vi "Update SyncMethod Events.vi"(8 "error in (no error)":errorcluster, 11 "Server class in":refnum<vi>) -> (0 "error out":errorcluster, 3 "Server class out":refnum<vi>)   [LabVIEW 2019, in "gRPC Scripting Tools.lvlib"]
uses:
  gRPC Scripting Tools.lvlib
  <vilib>/event_ctls.llb/lveventtype.ctl
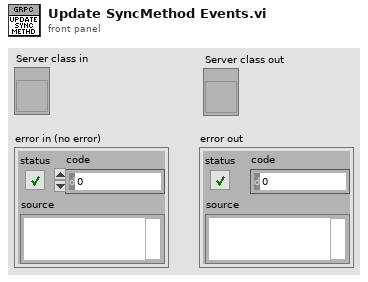
[diagram p1: front panel]
types:
  T1 = typedef "lveventtype.ctl" = enum32{"Null", "Timeout", "Annotation Menu Selection", "Annotation Menu Selection?", "App Instance Close", "App Instance Close?", "Autoscale Range Change", "Bookmark Info Change", "Cell Edit", "Cell Edit?", "Cursor Grab", "Cursor Grab?", "Cursor Menu Selection", "Cursor Menu Selection?", "Cursor Move", "Cursor Release", "Data Change", "Direction Change", "Display State Change", "Drag Ended", "Drag Enter", "Drag Leave", "Drag Over", "Drag Source Update", "Drag Starting", "Drag Starting?", "Drop", "Exec State Change", "Key Down", "Key Down?", "Key Repeat", "Key Repeat?", "Key Up", "Listbox Double Click", "Menu Activation?", "Menu Selection (App)", "Menu Selection? (App)", "Menu Selection (User)", "Mouse Down", "Mouse Down?", "Mouse Enter", "Mouse Leave", "Mouse Move", "Mouse Up", "Mouse Wheel", "NI Security User Change (App)", "Pane Size", "Panel Close", "Panel Close?", "Panel Resize", "Plot Attribute Change", "Scale Range Change", "Shortcut Menu Activation?", "Shortcut Menu Selection (App)", "Shortcut Menu Selection? (App)", "Shortcut Menu Selection (User)", "Tree Double Click", "Tree Drag", "Tree Drag?", "Tree Drop", "Tree Drop?", "Tree Item Close", "Tree Item Close?", "Tree Item Open", "Tree Item Open?", "User Event", "Value Change"}
  T2 = cluster{"Event Type":T1, "Event Registration Index":i32}
  T3 = cluster{"Event Type":T1, "Event Registration Index":i32}[]
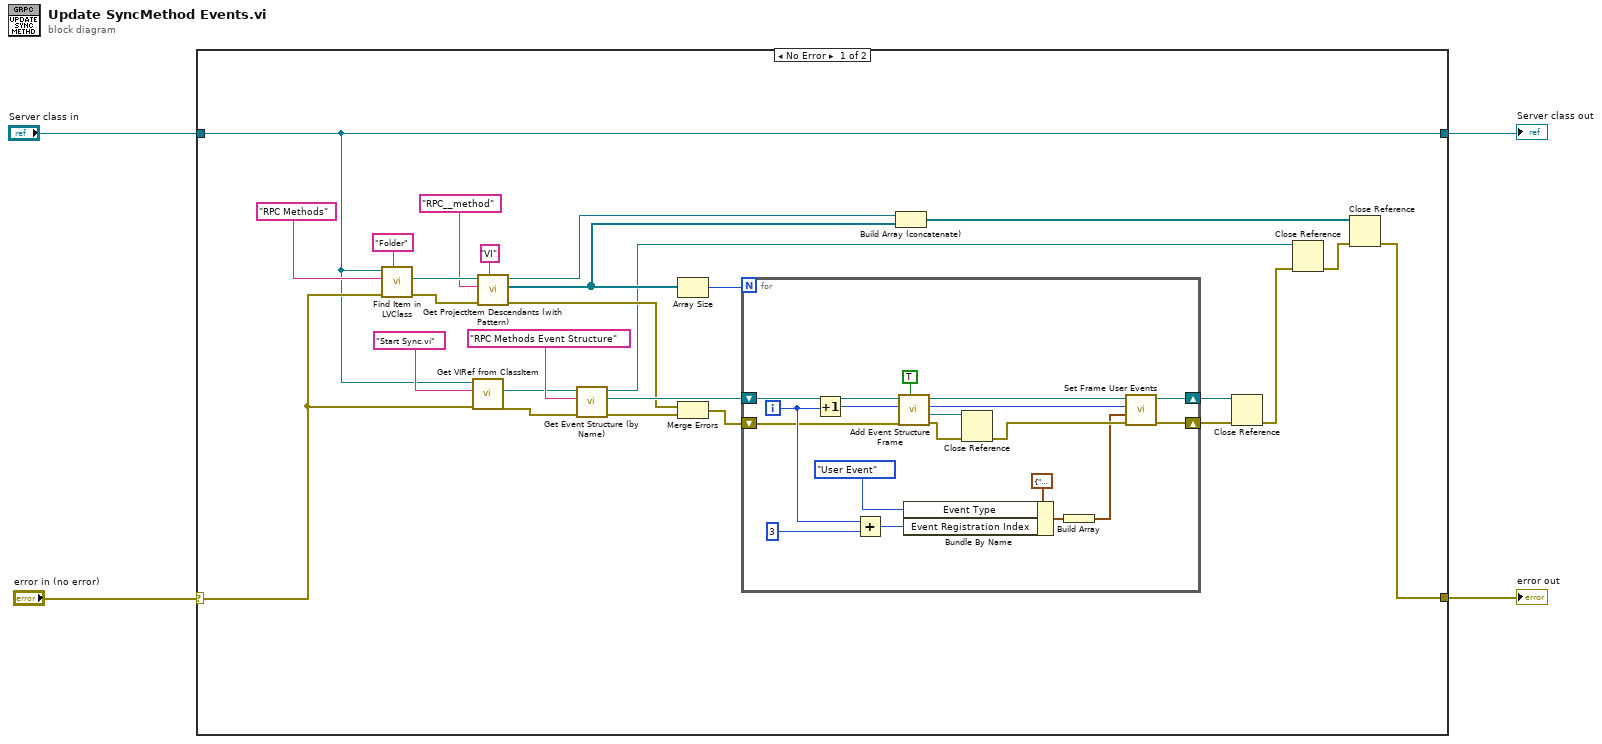
[diagram p0: block diagram]
diagram:
  n1 = case shown="No Error" "error in (no error)" {
    selector: "error in (no error)" -> [w6 w49]
    tunnel: "Server class in" -> [w5 w50]
    tunnel: [w7 w49] -> w3
    tunnel: [w5 w50] -> w1
    frame No Error {
      n2 = call "Find Item in LVClass.vi"("Item Type"="Folder", "error in (no error)"=w6, "Item Name"="RPC Methods", "Class Item in"=w5) -> ("error out"=w29:errorcluster, "Project Item (Class Item)"=w30:refnum<vi>)  [unwired: 4 in, 2 out]
      n3 = call "Get VIRef from ClassItem.vi"("error in (no error)"=w6, "Item Name"="Start Sync.vi", "LVClassLibrary in"=w5) -> ("error out"=w21:errorcluster, "VIref out"=w23:refnum<vi>)  [unwired: 5 in, 2 out]
      n4 = call "Get ProjectItem Descendants (with Pattern).vi"("Type"="VI", "error in (no error)"=w29, "Pattern"="RPC__method" ("regular expression"), "ProjectItem in"=w30) -> ("error out"=w13:errorcluster, "ProjectItem descendents"=w11:refnum<vi>[], "ProjectItem out"=w16:refnum<vi>)  [unwired: 5 in]
      n5 = call "Get Event Structure (by Name).vi"("error in (no error)"=w21, "Label"="RPC Methods Event Structure", "Owner VI in"=w23) -> ("error out"=w14:errorcluster, "Event Structure ref out"=w20:refnum<vi>, "Owner VI out"=w9:refnum<vi>)  [unwired: 5 in, 1 out]
      n6 = Array Size(array=w11) -> (size(s)=w19:i32)
      n7 = Merge Errors(w13, w14) -> (w12:errorcluster)
      n8 = for {
        N: w19 -> [_]
        shift-right: [w34] -> w18
        shift-left: w12 -> [w32]
        shift-right: [w31] -> w17
        shift-left: w20 -> [w33]
        i -> [w39]
        n9 = Increment(x=w39) -> (x+1=w42:i32)
        n10 = Add(x=w39, y=3) -> (x+y=w37:i32)
        n11 = call "Add Event Structure Frame.vi"("After? (T)"=TRUE, "error in (no error)"=w32, "Reference Frame Index"=w42, "Event Structure ref in"=w33) -> ("error out"=w48:errorcluster, "Added Frame"=w47:refnum<vi>, "Added Frame Index"=w45:i32, "Event Structure ref out"=w44:refnum<vi>)  [unwired: 4 in]
        n12 = Bundle By Name(cluster=T2 {"Event Type"=enum."User Event", "Event Registration Index"=3} ("Dynamic Events"), "Event Type"=lveventtype."User Event", "Event Registration Index"=w37) -> (w36:T2)
        n13 = Close Reference(reference=w47, error in (no error)=w48) -> (error out=w46:errorcluster)
        n14 = Build Array(w36) -> (w35:T3)
        n15 = call "Set Frame User Events.vi"("error in (no error)"=w46, "Dynamic Events"=w35, "Frame Index in"=w45, "Event Structure ref in"=w44) -> ("error out"=w34:errorcluster, "Event Structure ref out"=w31:refnum<vi>)  [unwired: 5 in, 1 out]
      }
      n16 = Build Array (concatenate)(w16, w11) -> (w15:refnum<vi>[])
      n17 = Close Reference(reference=w17, error in (no error)=w18) -> (error out=w10:errorcluster)
      n18 = Close Reference(reference=w9, error in (no error)=w10) -> (error out=w8:errorcluster)
      n19 = Close Reference(reference=w15, error in (no error)=w8) -> (error out=w7:errorcluster)
    }
    frame Error {
    }
  }
  "error out" <- w3
  "Server class out" <- w1
